vi "Scan SBlock Creator.vi"(8 "Common Parameters":T1[](array[typedef]), 9 "Number of repetitions":u16, 10 "Script Path":path, 11 "FPGA Name":string) -> (0 "error out":errorcluster, 2 "Schedule Block out":refnum<class "Schedule Block.lvclass">)   [LabVIEW 2020, in "CIRCUS_uServices.lvlib" / "Scheduler.lvlib" / "Scheduler.lvclass"]
uses:
  Scheduler.lvclass
  Scheduler.lvclass/Scheduler.ctl
  Run Utilities/Scan SBlock/Scan SBlock.lvclass
  Run Utilities/Run Instance/Run Instance.lvclass
  Run Utilities/Schedule Block/Schedule Block.lvclass
  Run Utilities/Schedule Block/Create SBlock (array of pairs).vi
  Run Utilities/Schedule/Schedule.lvclass
  Run Utilities/Scan SBlock/Parameter name with value - GUI.ctl
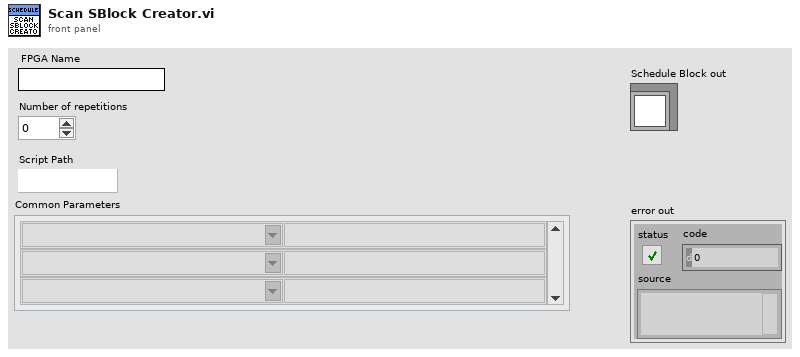
[diagram p1: front panel]
types:
  T1 = typedef "CIRCUS_uServices.lvlib/Run Utilities.lvlib/Scan SBlock.lvclass/Parameter name with value - GUI.ctl" = cluster{"Parameter Name":string, "Parameter Value":string}
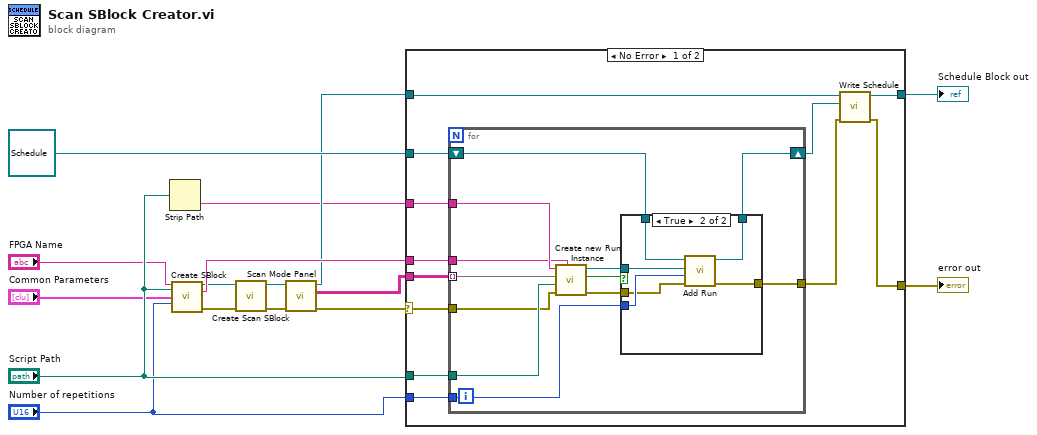
[diagram p0: block diagram]
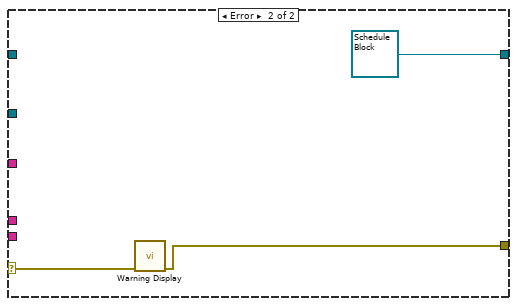
[diagram p3: hidden frame]
diagram:
  n1 = Strip Path(path="Script Path") -> (name=w1:string)  [unwired: 1 out]
  n2 = call-poly "Create SBlock.vi"("FPGA Name"="FPGA Name", "Script Path"="Script Path", "Common Parameters"="Common Parameters", "Number of repetitions"="Number of repetitions") -> ("Schedule Block out"=w9:refnum<class "Schedule Block.lvclass">, "FPGA Name"=w11:string, "error out"=w8:errorcluster)  [unwired: 9 in]
  n3 = call "Create Scan SBlock.vi"("error in (no error)"=w8, "Schedule Block in"=w9) -> ("error out"=w4:errorcluster, "Scan SBlock out"=w7:refnum<class "Scan SBlock.lvclass">)  [unwired: 8 in]
  n4 = call "Scan Mode Panel.vi"("error in (no error)"=w4, "Scan SBlock in"=w7) -> ("error out"=w5:errorcluster, "Parameters out"=w10:string[][][], "Schedule Block out"=w6:refnum<class "Schedule Block.lvclass">)  [unwired: 7 in]
  n5 = case shown="No Error" w5 {
    selector: w5 -> [w23 w50]
    tunnel: w1 -> [w28 _]
    tunnel: "Number of repetitions" -> [w27 _]
    tunnel: w10 -> [w26 _]
    tunnel: refnum<class "Schedule.lvclass"> refnum ("Run Tools.lvlib:Schedule.lvclass") -> [w25 _]
    tunnel: "Script Path" -> [w24 _]
    tunnel: [w19 w49] -> w3
    tunnel: [w22 refnum<class "Schedule Block.lvclass"> refnum ("Schedule Block out")] -> w14
    tunnel: w6 -> [w21 _]
    tunnel: w11 -> [w18 _]
    frame No Error {
      n6 = for {
        tunnel: w28 -> [w40]
        tunnel: w27 -> [w32]
        tunnel: w26 -> [w39] mode=indexing
        shift-right: [w34] -> w17
        shift-left: w25 -> [w35]
        tunnel: w24 -> [w38]
        tunnel: w23 -> [w37]
        tunnel: [w30] -> w20
        tunnel: w18 -> [w29]
        n7 = call "Create new Run Instance.vi"("Kasli"=w29, "error in"=w37, "Script Path"=w38, "Parameters"=w39, "Script Name"=w40) -> ("error out"=w31:errorcluster, "Created?"=w36:bool, "Run Instance"=w33:refnum<class "Run Instance.lvclass">)  [unwired: 4 in]
        n8 = case shown="True" w36 {
          tunnel: w35 -> [w42 w48]
          tunnel: [w42 w47] -> w34
          tunnel: w33 -> [_ w46]
          tunnel: w32 -> [_ w45]
          tunnel: w31 -> [w41 w44]
          tunnel: [w41 w43] -> w30
          frame False {
          }
          frame True {
            n9 = call-dynamic "Add Run.vi"("error in (no error)"=w44, "Number of repetitions"=w45, "Run Instance"=w46, "Schedule in"=w48) -> ("error out"=w43:errorcluster, "Schedule out"=w47:refnum<class "Schedule.lvclass">)  [unwired: 6 in]
          }
        }
      }
      n10 = call-dynamic "Write Schedule.vi"("error in (no error)"=w20, "Schedule"=w17, "Schedule Block in"=w21) -> ("error out"=w19:errorcluster, "Schedule Block out"=w22:refnum<class "Schedule Block.lvclass">)  [unwired: 7 in]
    }
    frame Error {
      n11 = call "Warning Display.vi"("error in (no error)"=w50) -> ("error out"=w49:errorcluster)  [unwired: 10 in]
    }
  }
  "error out" <- w3
  "Schedule Block out" <- w14
